vi "ContCheckCrystFluo.vi"(6 "FluoRef In":refnum<vi>, 8 "error in (no error)":errorcluster, 11 "readout":T1) -> (0 "error out":errorcluster, 3 "readout 2":T1, 5 "restart step?":bool)   [LabVIEW 2019]
uses:
  controls/FluoSettings.ctl
  <vilib>/Analysis/baseanly.llb/Mean (DBL).vi
  controls/GlobalExp.vi
  <vilib>/Analysis/NI_AALBase.lvlib
  Global.lvlib
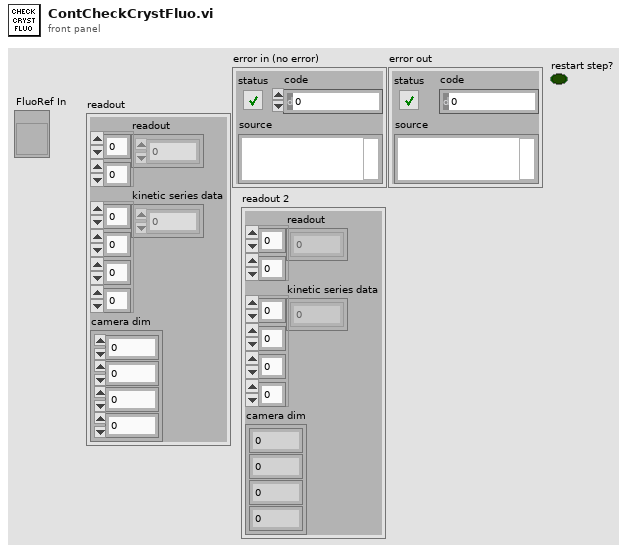
[diagram p1: front panel]
types:
  T1 = cluster{"readout":u32[][], "kinetic series data":i32[][][][], "camera dim":cluster{i32, i32, i32, i32}}
  T2 = typedef "MasterExpControl.ctl" = cluster{"Main Steps":dbl, "Main Runs":dbl, "ExpStatus":enum16{"Innit", "Stop", "Idle", "MainRunning", "AuxRunning"}, "Main Current Step":dbl, "ExpNum":dbl, "NewData":bool, "date":string, "command":string, "Stop":bool, "Pause":bool, "Mathematica":string, "Main/Meta":bool, "UpdateMath":bool, "Camera":bool, "MetaExpOver":bool, "NextMetaExp":bool}
  T3 = typedef "FluoSettings.ctl" = cluster{"Lock Fluorescence":bool, "Aux runs : ":i32, "Loop on test :":bool, "Loop frequency : ":bool, "Frequency Min":dbl, "Frequency Max":dbl, "PMT":cluster{"Lock point : ":dbl, "dF/dFl":dbl, "Unlock min":dbl, "Unlock max":dbl, "Loop min":dbl, "Loop max":dbl}, "Camera":cluster{"Lock point : ":dbl, "dF/dFl":dbl, "Unlock min":dbl, "Unlock max":dbl, "Loop min":dbl, "Loop max":dbl}}
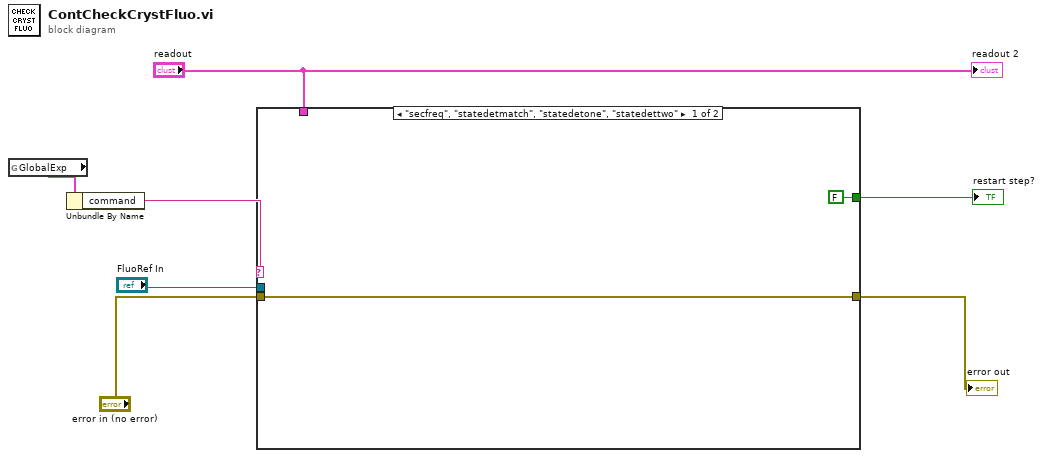
[diagram p0: block diagram]
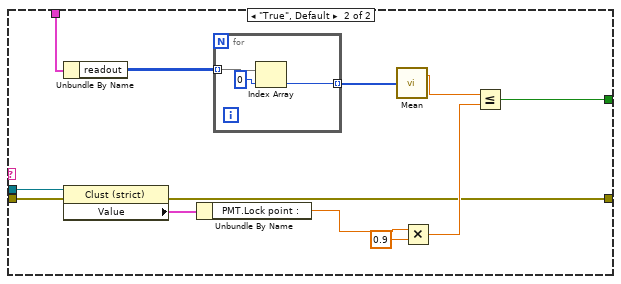
[diagram p2: hidden frame]
diagram:
  n1 = global read "GlobalExp.vi" "GlobalExp"() -> (w2:T2)
  n2 = Unbundle By Name(w2) -> ("command"=w1:string)
  n3 = case shown="\"secfreq\", \"statedetmatch\", \"statedetone\", \"statedettwo\"" w1 {
    tunnel: [FALSE w16] -> w7
    tunnel: "readout" -> [_ w15]
    tunnel: "FluoRef In" -> [_ w14]
    tunnel: "error in (no error)" -> [w8 w11]
    tunnel: [w8 w10] -> w3
    frame "secfreq", "statedetmatch", "statedetone", "statedettwo" {
    }
    frame "True", Default {
      n4 = Unbundle By Name(w15) -> ("readout"=w21:u32[][])
      n5 = property class="Clust (strict)"(reference=w14, error in=w11) -> (error out=w10:errorcluster, "Value"=w13:T3)  [unwired: 1 out]
      n6 = Unbundle By Name(w13) -> ("PMT.Lock point :"=w12:dbl)
      n7 = for {
        tunnel: w21 -> [w24] mode=indexing
        tunnel: [w22] -> w20 mode=indexing
        n8 = Index Array(array=w24, index=0) -> (element=w22:u32)
      }
      n9 = call-poly <vilib>:"Mean.vi"("X"=w20) -> ("mean"=w19:dbl)  [unwired: 1 out]
      n10 = Multiply(x=w12, y=0.9) -> (x*y=w17:dbl)
      n11 = Less Or Equal?(x=w19, y=w17) -> (x <= y?=w16:bool)
    }
  }
  "restart step?" <- w7
  "error out" <- w3
  "readout 2" <- "readout"
